vi "CheckAliasExists.vi"(9 "Alias":string, 10 "Actor":refnum<class "Actor.lvclass">) -> (2 "Error":errorcluster)   [LabVIEW 2020, in "jettl.lvlib"]
uses:
  jettl.lvlib
  Actor/Actor.lvclass
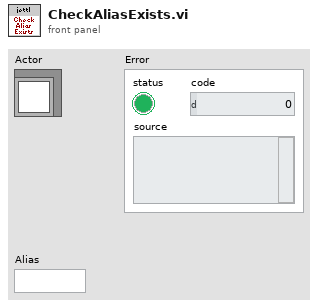
[diagram p1: front panel]
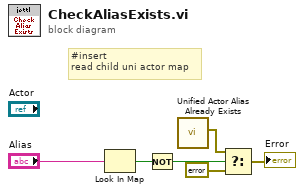
[diagram p0: block diagram]
diagram:
  # "#insert\nread child uni actor map"
  n1 = Look In Map(key="Alias") -> (map=w4:map{string, i32}, key not found?=w2:bool)  [unwired: 1 in, 1 out]
  n2 = Not(x=w2) -> (.not. x?=w1:bool)
  n3 = call "Unified Actor Alias Already Exists.vi"() -> ("Error"=w8:errorcluster)  [unwired: 11 in]
  n4 = Select(t=w8, s=w1, f=errorcluster {"status"=FALSE, "code"=0, "source"=""}) -> (s? t:f=→"Error":errorcluster)
